vi "Fouriersyntese.vi"() -> ()   [LabVIEW 2016]
uses:
  <vilib>/Analysis/2dsp.llb/Real FFT.vi
  <vilib>/measure/maspectr.llb/FFT Spectrum (Real-Im) for 1 Chan.vi
  <vilib>/measure/NI_MABase.lvlib
  <vilib>/measure/NI_MAPro.lvlib
  <vilib>/Analysis/NI_AALPro.lvlib
panel:
  in  "stop 2":bool
  out "signal out 4":dbl[](graph)
  out "signal out 3":waveform(ext)(graph)
  in  "No. of Coefficients":u16 step=1
  out "signal out 2":waveform(dbl)[](graph)=[{"t0"=timestamp(9.6 s since 1904-01-01), "dt"=0.0001, "Y"=array[3000 elements]}]
  out "signal out":waveform(dbl)(graph)={"t0"=timestamp(0 s since 1904-01-01), "dt"=0.0001, "Y"=array[3000 elements]}
  in  "Duty cycle [%]":dbl=50.0
  in  "Phase [Deg]":dbl min=0.0 max=360.0 step=30.0 format="%.0p"
  in  "Frequency":dbl=10.0 format="%.0p"
  in  "Signal Type":T1(ring)=enum."Square Wave"
  # "Fourier Synthesis"
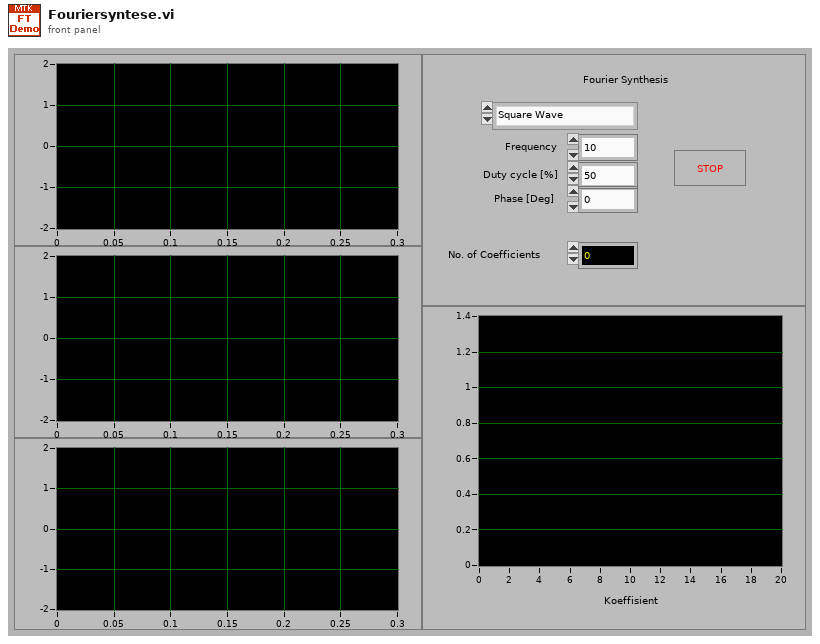
[diagram p1: front panel]
types:
  T1 = enum16{"Sine Wave", "Triangle Wave", "Square Wave", "Sawtooth Wave"}
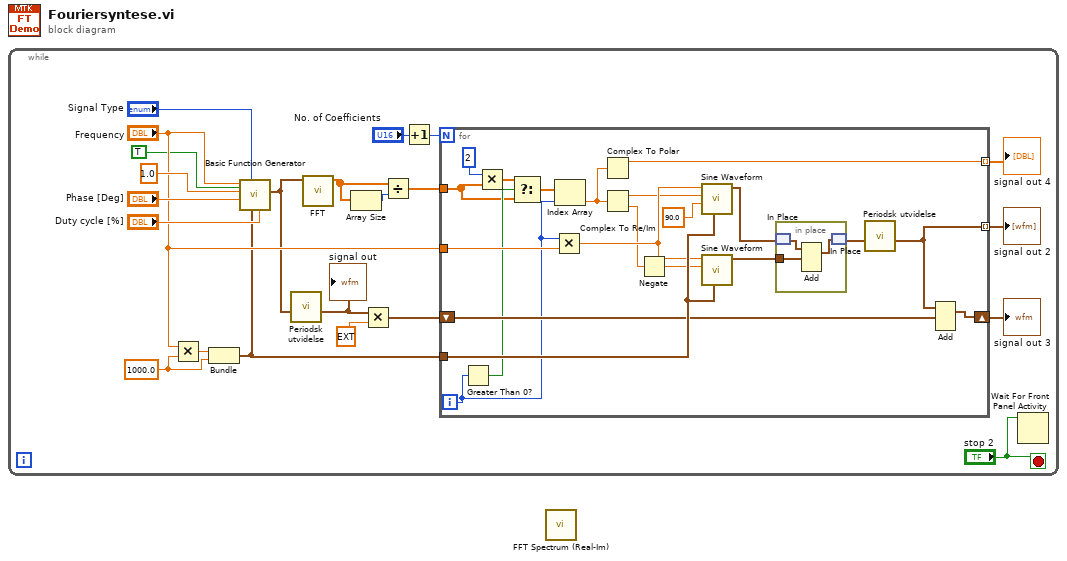
[diagram p0: block diagram]
diagram:
  n1 = while {
    stop <- "stop 2" stop-if-true
    w18 = 1000.0 ("#s")
    n2 = Multiply(x="Frequency", y=w18) -> (x*y=w17:dbl)
    n3 = Bundle(w17, "#s"=w18) -> (w15:cluster{dbl, "#s":dbl})  [unwired: 1 out]
    n4 = call <vilib>:"Basic Function Generator.vi"("square wave duty cycle (%)"="Duty cycle [%]", "reset signal"=TRUE, "sampling info"=w15, "signal type"="Signal Type", "phase"="Phase [Deg]", "amplitude"=1.0, "frequency"="Frequency") -> ("signal out"=w6:waveform(dbl))  [unwired: 2 in, 2 out]
    n5 = call "Periodsk utvidelse.vi"("Waveform in"=w6) -> ("Waveform out"=w2:waveform(dbl))  [unwired: 9 in, 1 out]
    "signal out" <- w2
    n6 = call-poly <vilib>:"FFT.vi"("X"=w6) -> ("FFT {X}"=w10:cdb[])  [unwired: 2 in, 8 out]
    n7 = Array Size(array=w10) -> (size(s)=w9:i32)
    n8 = Multiply(x=w2, y=ext 0.0 ("x")) -> (x*y=w4:waveform(ext))
    n9 = Divide(x=w10, y=w9) -> (x/y=w11:cdb[])
    n10 = Increment(x="No. of Coefficients") -> (x+1=w13:u16)
    n11 = for {
      N: w13 -> [_]
      tunnel: w11 -> [w26]
      tunnel: "Frequency" -> [w43]
      tunnel: w15 -> [w42]
      shift-right: [w36] -> w12
      shift-left: w4 -> [w38]
      tunnel: [w28] -> w8 mode=indexing
      tunnel: [w31] -> w7 mode=indexing
      i -> [w30]
      n12 = Greater Than 0?(x=w30) -> (x > 0?=w27:bool)
      n13 = Multiply(x=i16 2 ("y"), y=w26) -> (x*y=w24:cdb[])
      n14 = Select(t=w24, s=w27, f=w26) -> (s? t:f=w23:cdb[])
      n15 = Multiply(x=w30, y=w43) -> (x*y=w41:dbl)
      n16 = Index Array(array=w23, index=w30) -> (element=w34:cdb)
      n17 = Complex To Polar(r * e^(i*theta)=w34) -> (r=w31:dbl)  [unwired: 1 out]
      n18 = Complex To Re/Im(x + iy=w34) -> (x=w32:dbl, y=w35:dbl)
      n19 = Negate(x=w35) -> (-x=w33:dbl)
      n20 = call <vilib>:"Sine Waveform.vi"("sampling info"=w42, "phase"=90.0, "amplitude"=w32, "frequency"=w41) -> ("signal out"=w39:waveform(dbl))  [unwired: 3 in, 4 out]
      n21 = call <vilib>:"Sine Waveform.vi"("sampling info"=w42, "amplitude"=w33, "frequency"=w41) -> ("signal out"=w37:waveform(dbl))  [unwired: 4 in, 4 out]
      n22 = in-place {
        in-place-border: w37 -> [w45]
        n23 = in-place-match #1(w39) -> (w46:waveform(dbl))
        n24 = Add(1:w45, 2:w46) -> (0:w44:waveform(dbl))  [unwired: 1 in, 1 out]
        n25 = in-place-match #1(w44) -> (w29:waveform(dbl))
      }
      n26 = call "Periodsk utvidelse.vi"("Waveform in"=w29) -> ("Waveform out"=w28:waveform(dbl))  [unwired: 9 in, 1 out]
      n27 = Add(1:w38, 2:w28) -> (0:w36:waveform(ext))  [unwired: 1 in, 1 out]
    }
    "signal out 2" <- w8
    "signal out 3" <- w12
    "signal out 4" <- w7
    n28 = Wait For Front Panel Activity(3:"stop 2") -> ()  [unwired: 3 out]
  }
  n29 = call-poly <vilib>:"FFT Spectrum (Real-Im).vi"() -> ()  [unwired: 6 in, 6 out]
